vi "Read Instrument Data.vi"(7 "Slave Address":i32=-1 min=-1 max=30 step=1, 8 "error":errorcluster, 10 "Query":string, 11 "VISA":refnum<visa-resource-name>) -> (0 "error out":errorcluster, 1 "Return Count":u32, 2 "Response":string, 3 "VISA out":refnum<visa-resource-name>)   [LabVIEW 2019, in "TDK-Lambda GEN LAN Series.lvlib"]
doc: "Sends any SCPI query to the GEN and reads the response message. The Return Count is the number of characters read.\n\nIf a query error occurs, such as no response message because the query is illegal, the system error (SYST:ERR?) is read and returned in the \"error out\" cluster"
uses:
  <instrlib>/TDK-Lambda GEN LAN Series/TDK-Lambda GEN LAN Series.lvlib
panel:
  # "TDK-Lambda Genesys \n LAN\n  DC Power Supplies"
  # "Read Generic Query"
  # "Return any query errors"
  # "(Characters in response)"
  # "(c) 2019 TDK-Lambda.  ALL RIGHTS RESERVED."
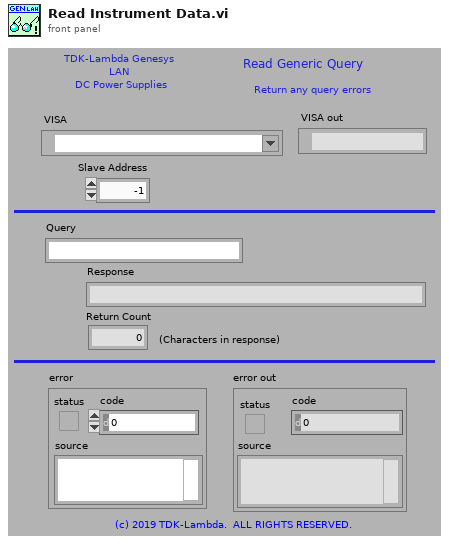
[diagram p1: front panel]
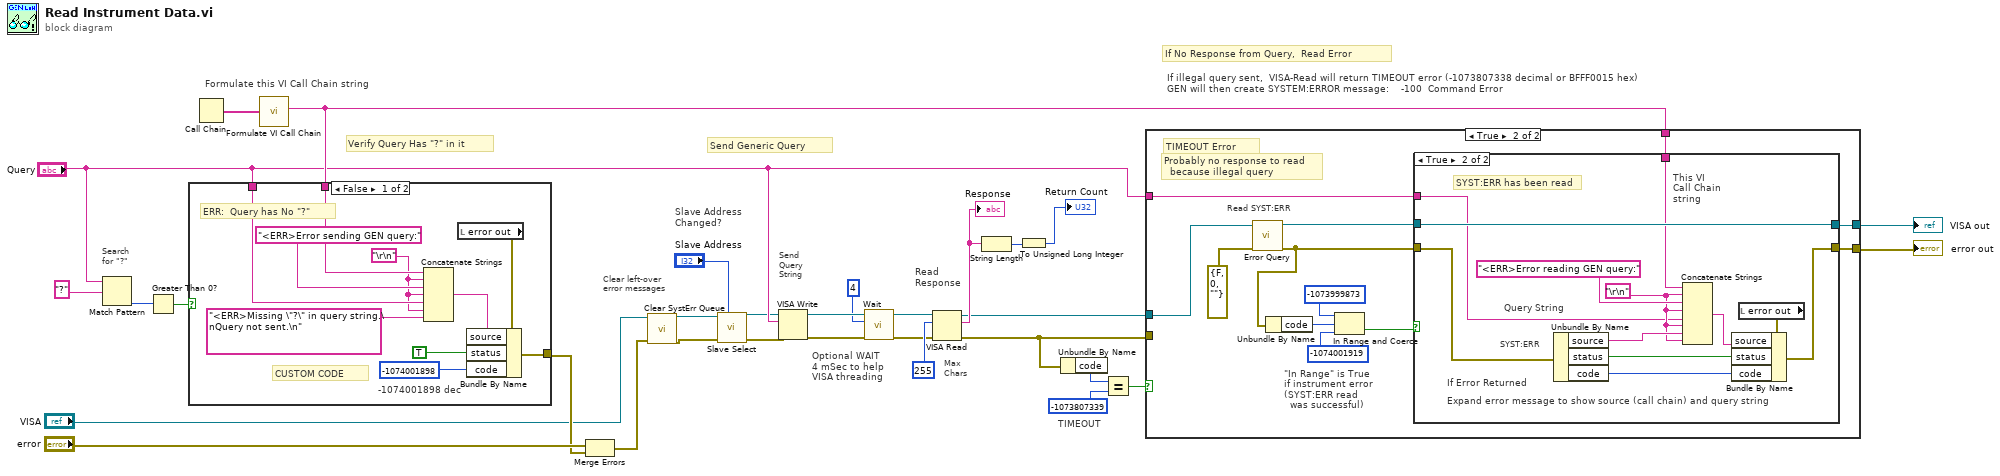
[diagram p0: block diagram]
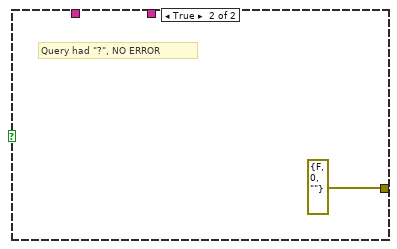
[diagram p2: hidden frame]
diagram:
  # "Optional WAIT \n4 mSec to help\nVISA threading"
  # "Clear left-over \nerror messages"
  # "Slave Address\nChanged?"
  # "Verify Query Has \"?\" in it"
  # "Read\nResponse"
  # "If No Response from Query,  Read Error"
  # "Send\nQuery\nString"
  # "Search\nfor \"?\""
  # "Formulate this VI Call Chain string"
  # "TIMEOUT"
  # "If illegal query sent,  VISA-Read will return TIMEOUT error (-1073807338 decimal or BFFF0015 hex) \nGEN will then create SYSTEM:ERROR message:    -100  Command Error"
  # "Max\nChars"
  # "Send Generic Query"
  n1 = Match Pattern(string="Query", regular expression="?") -> (offset past match=w22:i32)  [unwired: 1 in, 3 out]
  n2 = Greater Than 0?(x=w22) -> (x > 0?=w21:bool)
  n3 = Call Chain() -> (call chain=w17:string[])
  n4 = call <instrlib>:"Formulate VI Call Chain.vi"("Call Chain"=w17) -> ("String Out"=w16:string)  [unwired: 10 in]
  n5 = case shown="False" w21 {
    tunnel: w16 -> [w39 _]
    tunnel: "Query" -> [w37 _]
    tunnel: [w34 errorcluster {"status"=FALSE, "code"=0, "source"=""} ("error out")] -> w19
    frame False {
      w33 = "\r\n"
      # "-1074001898 dec"
      # "CUSTOM CODE"
      # "ERR:  Query has No \"?\""
      n6 = Concatenate Strings(w39, w33, "<ERR>Error sending GEN query:" ("Source"), w33, w37, w33, "<ERR>Missing \"?\" in query string.\nQuery not sent.\n" ("Source")) -> (w40:string)
      n7 = local read "error out"() -> (w41:errorcluster)
      n8 = Bundle By Name(cluster=w41, "source"=w40, "status"=TRUE, "code"=-1074001898) -> (w34:errorcluster)
    }
    frame True {
      # "Query had \"?\", NO ERROR"
    }
  }
  n9 = Merge Errors("error", w19) -> (w9:errorcluster)
  n10 = call <instrlib>:"Clear SystErr Queue.vi"("error"=w9, "VISA"="VISA") -> ("error out"=w10:errorcluster, "VISA out"=w12:refnum<visa-resource-name>)  [unwired: 8 in]
  n11 = call <instrlib>:"Slave Select.vi"("Slave Address"="Slave Address", "error"=w10, "VISA"=w12) -> ("error out"=w13:errorcluster, "VISA out"=w14:refnum<visa-resource-name>)  [unwired: 7 in]
  n12 = VISA Write(VISA resource name=w14, write buffer="Query", error in (no error)=w13) -> (VISA resource name out=w6:refnum<visa-resource-name>, error out=w4:errorcluster)  [unwired: 1 out]
  n13 = call <instrlib>:"Wait.vi"("error"=w4, "Delay (20 mS)"=u32 4, "VISA"=w6) -> ("error out"=w3:errorcluster, "VISA out"=w5:refnum<visa-resource-name>)  [unwired: 7 in]
  n14 = VISA Read(VISA resource name=w5, byte count=u32 255 ("byte count (0)"), error in (no error)=w3) -> (VISA resource name out=w8:refnum<visa-resource-name>, read buffer=w18:string, error out=w7:errorcluster)  [unwired: 1 out]
  "Response" <- w18
  n15 = String Length(string=w18) -> (length=w29:i32)
  n16 = To Unsigned Long Integer(number=w29) -> (unsigned 32bit integer=→"Return Count":u32)
  n17 = Unbundle By Name(w7) -> ("code"=w25:i32)
  n18 = Equal?(x=w25, y=-1073807339 ("code")) -> (x = y?=w27:bool)
  n19 = case shown="True" w27 {
    tunnel: [w43 w55] -> w24
    tunnel: [w44 w56] -> w31
    tunnel: w8 -> [w44 w49]
    tunnel: w7 -> [w43 _]
    tunnel: w16 -> [_ w46]
    tunnel: "Query" -> [_ w45]
    frame False {
      # "Maybe some other VISA error,  pass it out\nIf error occurred, , \"Response\" is empty and \"Return Count\" is zero"
      # "Not TIMEOUT Error (maybe successful query)"
    }
    frame True {
      # "\"In Range\" is True\nif instrument error\n(SYST:ERR read\n  was successful)"
      # "TIMEOUT Error"
      # "Probably no response to read  \n  because illegal query"
      # "Read SYST:ERR"
      n20 = call <instrlib>:"Error Query.vi"("error"=errorcluster {"status"=FALSE, "code"=0, "source"=""}, "VISA"=w49) -> ("error out"=w48:errorcluster, "VISA out"=w47:refnum<visa-resource-name>)  [unwired: 6 in, 2 out]
      n21 = Unbundle By Name(w48) -> ("code"=w51:i32)
      n22 = In Range and Coerce(upper limit=-1073999873 ("code"), x=w51, lower limit=-1074001919 ("code")) -> (In Range?=w52:bool)  [unwired: 1 out]
      n23 = case shown="True" w52 {
        tunnel: w48 -> [w58 w63]
        tunnel: [w58 w64] -> w55
        tunnel: w47 -> [w57 w62]
        tunnel: [w57 w62] -> w56
        tunnel: w46 -> [_ w60]
        tunnel: w45 -> [_ w59]
        frame False {
          # "Read SYST:ERR returned VISA communication error.\n  Comm is dead,  just pass error out"
        }
        frame True {
          w61 = "\r\n"
          # "Query String"
          # "Expand error message to show source (call chain) and query string"
          # "This VI \nCall Chain \nstring"
          # "SYST:ERR"
          # "If Error Returned"
          # "SYST:ERR has been read"
          n24 = Unbundle By Name(w63) -> ("source"=w67:string, "status"=w69:bool, "code"=w68:i32)
          n25 = Concatenate Strings(w60, w61, "<ERR>Error reading GEN query:" ("Source"), w61, w59, w61, w67, w61) -> (w70:string)
          n26 = local read "error out"() -> (w65:errorcluster)
          n27 = Bundle By Name(cluster=w65, "source"=w70, "status"=w69, "code"=w68) -> (w64:errorcluster)
        }
      }
    }
  }
  "VISA out" <- w31
  "error out" <- w24
